vi "Get Adjascent.vi"(8 "Side":T1, 9 "Column In":i32, 10 "Row In":i32, 11 "Array In":i32[][](array[numeric])) -> (1 "Column Out":i32[](array[numeric]), 2 "Row Out":i32[](array[numeric]), 3 "Array":i32[](array[numeric]))   [LabVIEW 2019]
uses:
  Day 11/Controls/Side.ctl
  Day 11/Day 11.lvlib
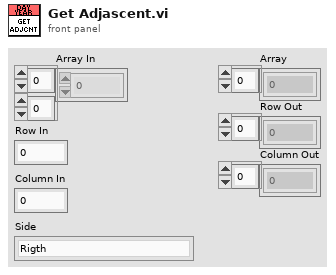
[diagram p1: front panel]
types:
  T1 = typedef "Day 11.lvlib/Side.ctl" = enum16{"Rigth", "Left", "Down", "Up", "Rigth Up", "Rigth Down", "Left Up", "Left Down"}
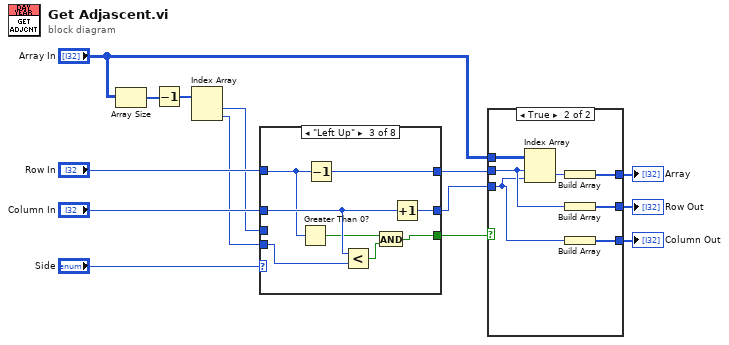
[diagram p0: block diagram]
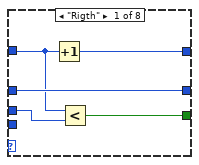
[diagram p2: hidden frame]
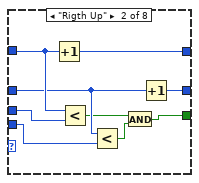
[diagram p3: hidden frame]
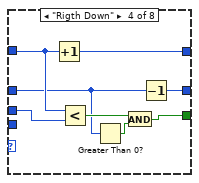
[diagram p4: hidden frame]
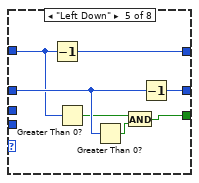
[diagram p5: hidden frame]
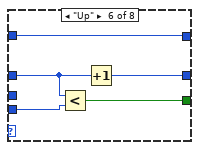
[diagram p6: hidden frame]
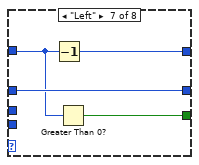
[diagram p7: hidden frame]
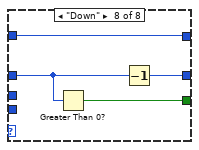
[diagram p8: hidden frame]
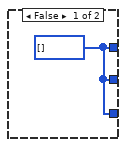
[diagram p9: hidden frame]
diagram:
  n1 = Array Size(array="Array In") -> (size(s)=w13:i32[])
  n2 = Decrement(x=w13) -> (x-1=w12:i32[])
  n3 = Index Array(array=w12) -> (element #1=w5:i32, element #2=w4:i32)  [unwired: 2 in]
  n4 = case shown="\"Left Up\"" "Side" {
    tunnel: "Row In" -> [w17 w27 w30 w43 w46 w56 w58 w64]
    tunnel: "Column In" -> [w19 w24 w35 w38 w49 w53 w60 w62]
    tunnel: [w19 w25 w36 w41 w51 w52 w60 w61] -> w6
    tunnel: [w18 w28 w31 w44 w47 w56 w59 w64] -> w7
    tunnel: w5 -> [w16 w26 _ w42 _ _ _ _]
    tunnel: w4 -> [_ w23 w34 _ _ w54 _ _]
    tunnel: [w15 w20 w32 w39 w50 w55 w57 w63] -> w3
    frame "Rigth" {
      n5 = Increment(x=w17) -> (x+1=w18:i32)
      n6 = Less?(x=w17, y=w16) -> (x < y?=w15:bool)
    }
    frame "Rigth Up" {
      n7 = Increment(x=w27) -> (x+1=w28:i32)
      n8 = Less?(x=w27, y=w26) -> (x < y?=w22:bool)
      n9 = Less?(x=w24, y=w23) -> (x < y?=w21:bool)
      n10 = And(x=w22, y=w21) -> (x .and. y?=w20:bool)
      n11 = Increment(x=w24) -> (x+1=w25:i32)
    }
    frame "Left Up" {
      n12 = Greater Than 0?(x=w30) -> (x > 0?=w29:bool)
      n13 = Decrement(x=w30) -> (x-1=w31:i32)
      n14 = Less?(x=w35, y=w34) -> (x < y?=w33:bool)
      n15 = And(x=w29, y=w33) -> (x .and. y?=w32:bool)
      n16 = Increment(x=w35) -> (x+1=w36:i32)
    }
    frame "Rigth Down" {
      n17 = Increment(x=w43) -> (x+1=w44:i32)
      n18 = Less?(x=w43, y=w42) -> (x < y?=w40:bool)
      n19 = Greater Than 0?(x=w38) -> (x > 0?=w37:bool)
      n20 = And(x=w40, y=w37) -> (x .and. y?=w39:bool)
      n21 = Decrement(x=w38) -> (x-1=w41:i32)
    }
    frame "Left Down" {
      n22 = Decrement(x=w46) -> (x-1=w47:i32)
      n23 = Greater Than 0?(x=w46) -> (x > 0?=w45:bool)
      n24 = Greater Than 0?(x=w49) -> (x > 0?=w48:bool)
      n25 = And(x=w45, y=w48) -> (x .and. y?=w50:bool)
      n26 = Decrement(x=w49) -> (x-1=w51:i32)
    }
    frame "Up" {
      n27 = Less?(x=w53, y=w54) -> (x < y?=w55:bool)
      n28 = Increment(x=w53) -> (x+1=w52:i32)
    }
    frame "Left" {
      n29 = Decrement(x=w58) -> (x-1=w59:i32)
      n30 = Greater Than 0?(x=w58) -> (x > 0?=w57:bool)
    }
    frame "Down" {
      n31 = Greater Than 0?(x=w62) -> (x > 0?=w63:bool)
      n32 = Decrement(x=w62) -> (x-1=w61:i32)
    }
  }
  n33 = case shown="True" w3 {
    tunnel: w7 -> [_ w69]
    tunnel: "Array In" -> [_ w72]
    tunnel: w6 -> [_ w68]
    tunnel: [w65 w70] -> w14
    tunnel: [w65 w67] -> w1
    tunnel: [w65 w66] -> w2
    frame False {
      w65 = i32[] []
    }
    frame True {
      n34 = Index Array(array=w72, index (row)=w69, index (col)=w68) -> (element=w71:i32)
      n35 = Build Array(w71) -> (w70:i32[])
      n36 = Build Array(w69) -> (w67:i32[])
      n37 = Build Array(w68) -> (w66:i32[])
    }
  }
  "Array" <- w14
  "Row Out" <- w1
  "Column Out" <- w2
